vi "drive2.vi"(9 "Distance (cm)":dbl) -> ()   [LabVIEW 2014, in "Janga.lvrbt"]
uses:
  Janga.lvrbt
  <vilib>/NXT/Block Support/NXT_OutputPort.ctl
  <vilib>/NXT/NXTIO Xnodes/NXTIONodeSubVIs/LEGOMotorStatus.vi
  <vilib>/NXT/NXTIO Xnodes/NXTIONodeSubVIs/NXTMoveMotors.vi
  <vilib>/NXT/NXTIO Xnodes/NXTIONodeSubVIs/NXTStopMotors.vi
  <vilib>/NXT/NXTIO Xnodes/NXTIONodeSubVIs/LEGOResetMotors.vi
  <vilib>/NXT/NXTIO Xnodes/AddressXNode/NXTIOAddress.xnode
  <vilib>/NXT/Subs/LVHSConnector.ctl
  <vilib>/NXT/NXTIO Xnodes/NXTIOXNode/NXTIO.xnode
  <vilib>/NXT/LegoClasses/BrickReference/BrickReference.lvclass
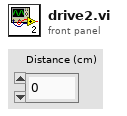
[diagram p1: front panel]
types:
  T1 = typedef "NXT_OutputPort.ctl" = u8
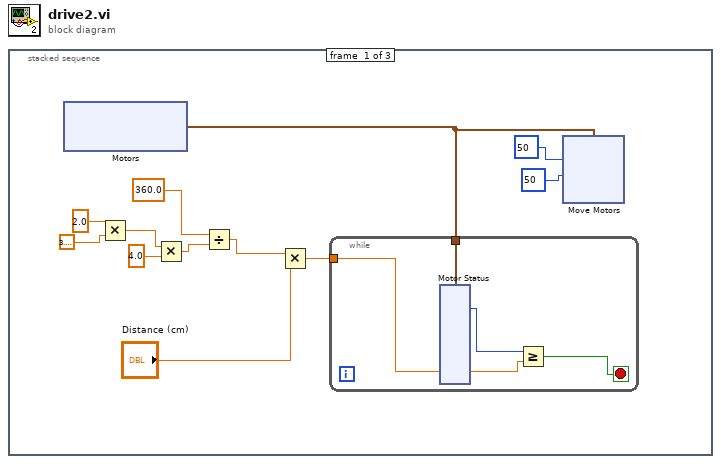
[diagram p0: block diagram]
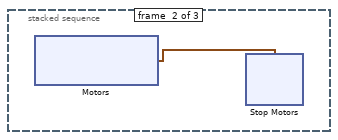
[diagram p2: hidden frame]
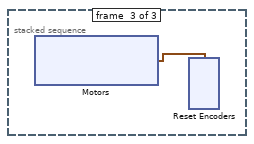
[diagram p3: hidden frame]
diagram:
  n1 = stacked-sequence {
    frame #0 {
      n2 = xnode "Motors"() -> ("Motor"=w2:cluster{"Port":T1, "Port":T1})
      n3 = Multiply(x=2.0, y=3.141592653589793) -> (x*y=w7:dbl)
      n4 = Multiply(x=w7, y=4.0) -> (x*y=w6:dbl)
      n5 = Divide(x=360.0, y=w6) -> (x/y=w11:dbl)
      n6 = Multiply(x=w11, y="Distance (cm)") -> (x*y=w4:dbl)
      n7 = while {
        tunnel: w4 -> [w24]
        tunnel: w2 -> [w22]
        stop <- w23 stop-if-true
        n8 = xnode "Motor Status"("Motors"=w22) -> ("Position 1"=w25:i32)  [unwired: 1 in, 4 out]
        n9 = Greater Or Equal?(x=w25, y=w24) -> (x >= y?=w23:bool)
      }
      n10 = xnode "Move Motors"("Power/Speed 2"=i8 50, "Power/Speed 1"=i8 50, "Motors"=w2) -> ()  [unwired: 1 in, 1 out]
    }
    frame #1 {
      n11 = xnode "Motors"() -> ("Motor"=w36:cluster{"Port":T1, "Port":T1})
      n12 = xnode "Stop Motors"("Motors"=w36) -> ()  [unwired: 1 in, 1 out]
    }
    frame #2 {
      n13 = xnode "Motors"() -> ("Motor"=w43:cluster{"Port":T1, "Port":T1})
      n14 = xnode "Reset Encoders"("Motors"=w43) -> ()  [unwired: 1 in, 1 out]
    }
  }
